vi "CSMLS - Append Continious State.vi"(6 "Loop State(s) and Arguments":string, 9 "Continous Arguments (\"\")":string, 10 "Continous State":string, 11 "Remaining States":string) -> (3 "States Out":string)   [LabVIEW 2014, in "CSM Loop Support.lvlib"]
uses:
  CSM Loop Support.lvlib
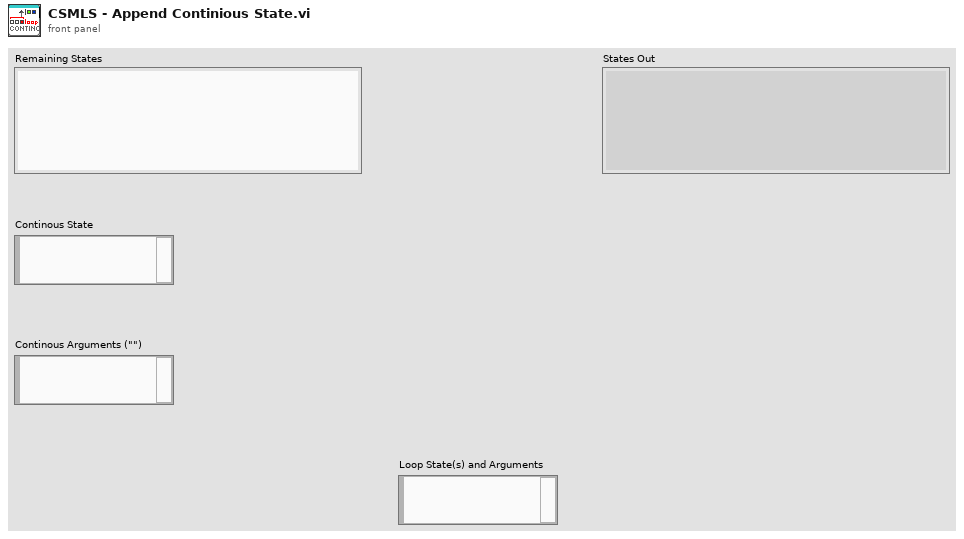
[diagram p1: front panel]
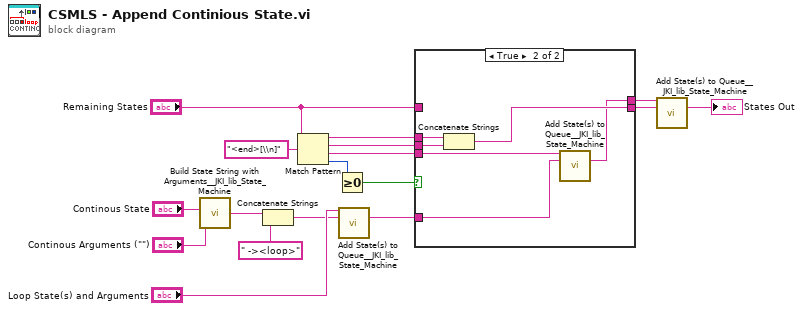
[diagram p0: block diagram]
diagram:
  n1 = call <vilib>:"Build State String with Arguments__JKI_lib_State_Machine.vi"("Arguments (\"\")"="Continous Arguments (\"\")", "State"="Continous State") -> ("State with Arguments"=w14:string)  [unwired: 4 in]
  n2 = Concatenate Strings(w14, " -><loop>" ("string")) -> (w12:string)
  n3 = Match Pattern(string="Remaining States", regular expression="<end>[\\n]") -> (before substring=w5:string, match substring=w4:string, after substring=w3:string, offset past match=w9:i32)  [unwired: 1 in]
  n4 = Greater Or Equal To 0?(x=w9) -> (x >= 0?=w8:bool)
  n5 = call <vilib>:"Add State(s) to Queue__JKI_lib_State_Machine.vi"("State(s) in Front (\"\")"="Loop State(s) and Arguments", "State(s) in (\"\")"=w12) -> ("States Out"=w1:string)  [unwired: 13 in]
  n6 = case shown="True" w8 {
    tunnel: [w19 w23] -> w7
    tunnel: "Remaining States" -> [w19 _]
    tunnel: w5 -> [_ w25]
    tunnel: w4 -> [_ w24]
    tunnel: w3 -> [_ w22]
    tunnel: [w18 w20] -> w2
    tunnel: w1 -> [w18 w21]
    frame False {
    }
    frame True {
      n7 = Concatenate Strings(w25, w24) -> (w23:string)
      n8 = call <vilib>:"Add State(s) to Queue__JKI_lib_State_Machine.vi"("State(s) in Front (\"\")"=w22, "State(s) in (\"\")"=w21) -> ("States Out"=w20:string)  [unwired: 13 in]
    }
  }
  n9 = call <vilib>:"Add State(s) to Queue__JKI_lib_State_Machine.vi"("State(s) in Front (\"\")"=w2, "State(s) in (\"\")"=w7) -> ("States Out"=→"States Out":string)  [unwired: 13 in]
